vi "Back.vi"(0 "reference in":refnum<class "Slide.lvclass">, 5 "error in (no error)":errorcluster) -> (14 "reference out":refnum<class "Slide.lvclass">, 19 "error out":errorcluster)   [LabVIEW 2013, in "Slide.lvclass"]
uses:
  Slide.lvclass
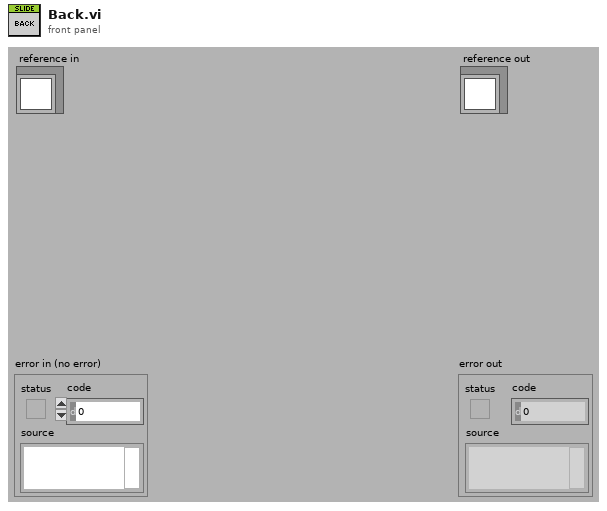
[diagram p1: front panel]
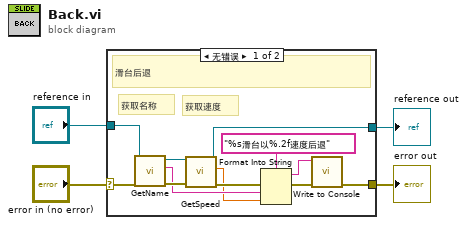
[diagram p0: block diagram]
diagram:
  n1 = case shown="无错误" "error in (no error)" {
    selector: "error in (no error)" -> [w10 w18]
    tunnel: [w11 w18] -> w3
    tunnel: [w12 w17] -> w1
    tunnel: "reference in" -> [w8 w17]
    frame No Error {
      # "获取速度"
      # "获取名称"
      # "滑台后退"
      n2 = call-dynamic "GetName.vi"("error in (no error)"=w10, "reference in"=w8) -> ("error out"=w9:errorcluster, "Name"=w6:string, "reference out"=w7:refnum<class "Slide.lvclass">)  [unwired: 7 in]
      n3 = call-dynamic "GetSpeed.vi"("error in (no error)"=w9, "reference in"=w7) -> ("error out"=w13:errorcluster, "Speed"=w5:dbl, "reference out"=w12:refnum<class "Slide.lvclass">)  [unwired: 7 in]
      n4 = Format Into String(format string="%s滑台以%.2f速度后退" ("Input"), error in=w13, w6, w5) -> (resulting string=w15:string, error out=w16:errorcluster)  [unwired: 1 in]
      n5 = call "Write to Console.vi"("error in (no error)"=w16, "Input"=w15) -> ("error out"=w11:errorcluster)  [unwired: 9 in]
    }
    frame Error {
    }
  }
  "error out" <- w3
  "reference out" <- w1
